vi "Check Password.vi"(8 "error in (no error)":errorcluster) -> (0 "error out":errorcluster, 3 "Valid?":bool)   [LabVIEW 2015]
panel:
  out "Misses":dbl
  in  "Cancel":bool
  in  "Continue":bool
  in  "Password":string
  in  "Username":string
  # "Please type in your username and password"
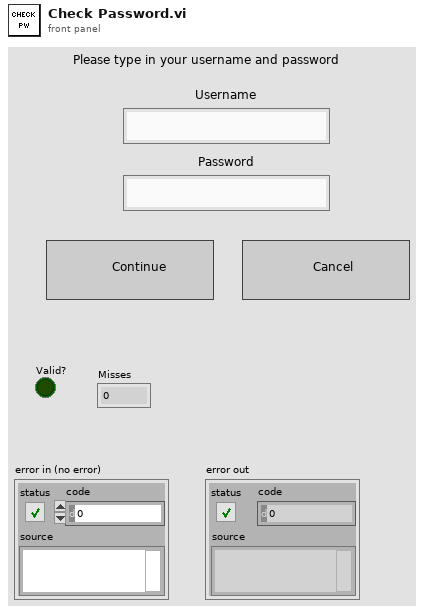
[diagram p1: front panel]
types:
  T1 = typedef "LVPositionTypeDef.ctl" = cluster{"Left":i32, "Top":i32}
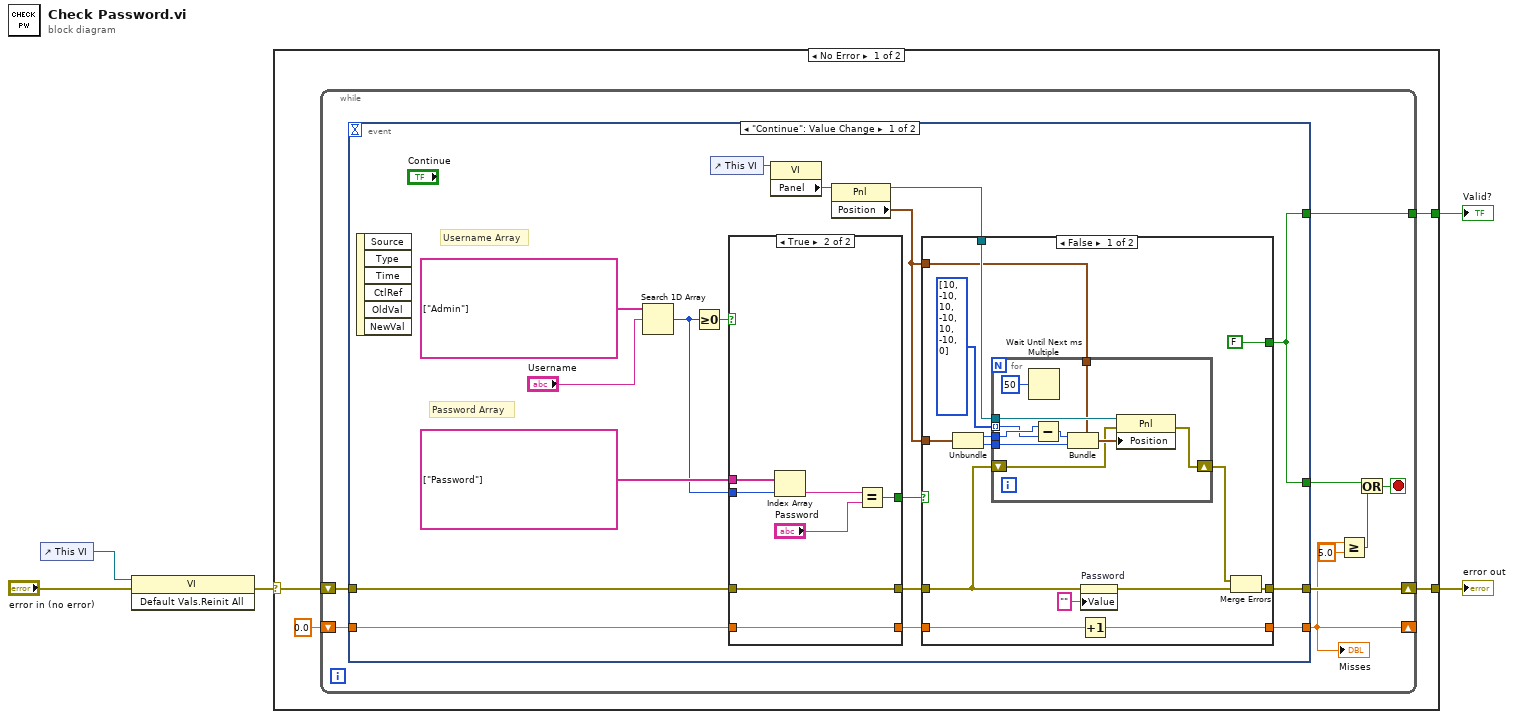
[diagram p0: block diagram]
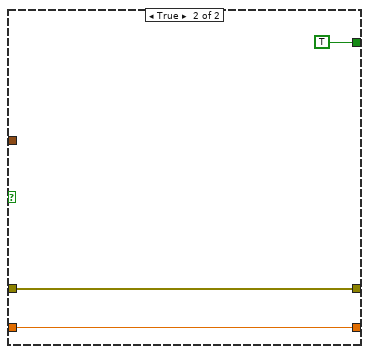
[diagram p2: hidden frame]
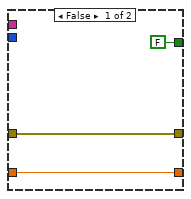
[diagram p3: hidden frame]
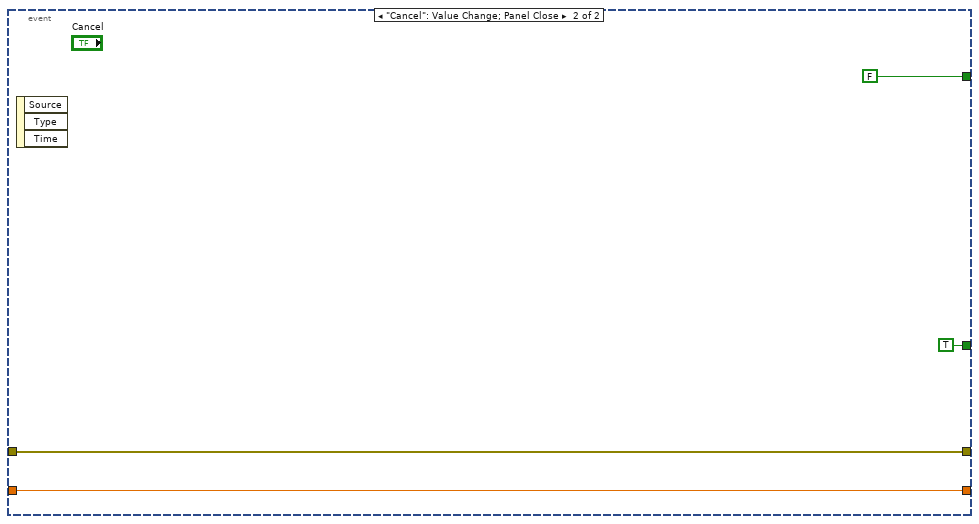
[diagram p4: hidden frame]
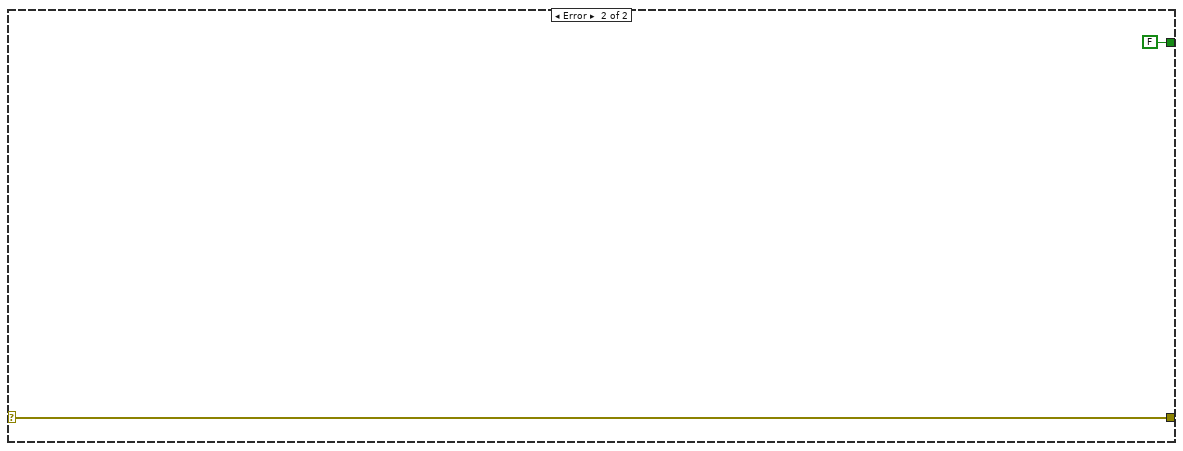
[diagram p5: hidden frame]
diagram:
  n1 = control-ref of="This VI"() -> (w2:refnum<vi>)
  n2 = invoke class="VI" method="Default Vals.Reinit All"(reference=w2, error in="error in (no error)") -> (error out=w3:errorcluster)  [unwired: 1 in, 2 out]
  n3 = case shown="No Error" w3 {
    selector: w3 -> [w9 w78]
    tunnel: [w8 w78] -> w5
    tunnel: [w7 FALSE] -> w4
    frame No Error {
      n4 = while {
        shift-right: [w17] -> w8
        shift-left: w9 -> [w18]
        tunnel: [w15] -> w7
        shift-right: [w12] -> _
        shift-left: 0.0 -> [w14]
        stop <- w11 stop-if-true
        n5 = event shown="[0] \"Continue\": Value Change" {
          selector: _ -> [_ _]
          dyn-events: _ -> [_ _]
          timeout: _ -> [_ _]
          tunnel: w18 -> [w29 w74]
          tunnel: [w27 w74] -> w17
          tunnel: [w26 FALSE] -> w15
          tunnel: [w26 TRUE] -> w16
          tunnel: [w22 w73] -> w12
          tunnel: w14 -> [w21 w73]
          event "Continue": Value Change {
            # "Password Array"
            # "Username Array"
            n6 = event-data() -> ()  [unwired: 1 in, 6 out]
            n7 = Search 1D Array(1D array=string[] ["Admin"], element="Username") -> (index of element=w31:i32)  [unwired: 1 in]
            n8 = Greater Or Equal To 0?(x=w31) -> (x >= 0?=w33:bool)
            n9 = control-ref of="This VI"() -> (w25:refnum<vi>)
            n10 = case shown="True" w33 {
              tunnel: string[] ["Password"] -> [_ w72]
              tunnel: w31 -> [_ w71]
              tunnel: [FALSE w68] -> w30
              tunnel: w29 -> [w65 w67]
              tunnel: [w65 w67] -> w28
              tunnel: w21 -> [w63 w66]
              tunnel: [w63 w66] -> w20
              frame False {
              }
              frame True {
                n11 = Index Array(array=w72, index=w71) -> (element=w70:string)
                n12 = Equal?(x=w70, y="Password") -> (x = y?=w68:bool)
              }
            }
            n13 = property class="VI"(reference=w25) -> ("Panel"=w24:refnum<vi>)  [unwired: 1 in, 2 out]
            n14 = property class="Pnl"(reference=w24) -> (reference out=w23:refnum<vi>, "Position"=w19:T1)  [unwired: 1 in, 1 out]
            n15 = case shown="False" w30 {
              tunnel: [FALSE TRUE] -> w26
              tunnel: w28 -> [w43 w62]
              tunnel: [w41 w62] -> w27
              tunnel: w19 -> [w49 _]
              tunnel: w23 -> [w47 _]
              tunnel: [w38 w60] -> w22
              tunnel: w20 -> [w37 w60]
              tunnel: w19 -> [w36 _]
              frame False {
                n16 = Unbundle(w49) -> ("Left"=w48:i32, "Top"=w46:i32)
                n17 = for {
                  tunnel: w48 -> [w53]
                  tunnel: w47 -> [w59]
                  tunnel: w46 -> [w58]
                  tunnel: w36 -> [w56]
                  shift-right: [w54] -> w40
                  shift-left: w43 -> [w55]
                  tunnel: i32[] [10, -10, 10, -10, 10, -10, 0] -> [w51] mode=indexing
                  n18 = Wait Until Next ms Multiple(millisecond multiple=u32 50) -> ()  [unwired: 1 out]
                  n19 = Subtract(x=w53, y=w51) -> (x-y=w52:i32)
                  n20 = Bundle(cluster=w56, "Left"=w52, "Top"=w58) -> (w57:T1)
                  n21 = property class="Pnl"(reference=w59, error in=w55, "Position"=w57) -> (error out=w54:errorcluster)  [unwired: 1 out]
                }
                n22 = Increment(x=w37) -> (x+1=w38:dbl)
                n23 = property on="Password" class="Str"(error in=w43, "Value"="" ("Password")) -> (error out=w42:errorcluster)  [unwired: 1 in, 1 out]
                n24 = Merge Errors(w40, w42) -> (w41:errorcluster)
              }
              frame True {
              }
            }
          }
          event "Cancel": Value Change; Panel Close {
            n25 = event-data() -> ()  [unwired: 1 in, 3 out]
          }
        }
        "Misses" <- w12
        n26 = Greater Or Equal?(x=w12, y=5.0) -> (x >= y?=w10:bool)
        n27 = Or(x=w16, y=w10) -> (x .or. y?=w11:bool)
      }
    }
    frame Error {
    }
  }
  "error out" <- w5
  "Valid?" <- w4
